vi "Write Common Parameters.vi"(8 "error in (no error)":errorcluster, 10 "Common Parameters":string[][](array[string]), 11 "Schedule Block in":refnum<class "Schedule Block.lvclass">) -> (0 "error out":errorcluster, 3 "Schedule Block out":refnum<class "Schedule Block.lvclass">)   [LabVIEW 2020, in "Run Utilities.lvlib" / "Schedule Block.lvclass"]
uses:
  Schedule Block.lvclass
  Schedule Block.lvclass/Schedule Block.ctl
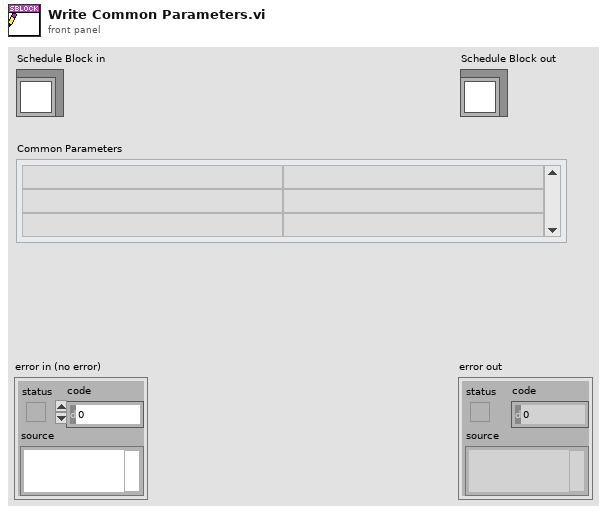
[diagram p1: front panel]
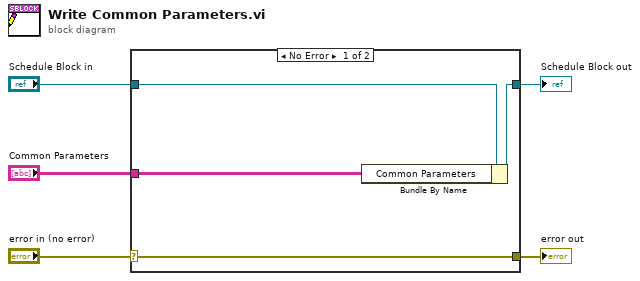
[diagram p0: block diagram]
diagram:
  n1 = case shown="No Error" "error in (no error)" {
    selector: "error in (no error)" -> [w9 w10]
    tunnel: [w9 w10] -> w4
    tunnel: [w7 w11] -> w2
    tunnel: "Schedule Block in" -> [w8 w11]
    tunnel: "Common Parameters" -> [w6 _]
    frame No Error {
      n2 = Bundle By Name(cluster=w8, "Common Parameters"=w6) -> (w7:refnum<class "Schedule Block.lvclass">)
    }
    frame Error {
    }
  }
  "error out" <- w4
  "Schedule Block out" <- w2
